vi "Guys Version Host.vi"() -> ()   [LabVIEW 2014]
uses:
  <instrlib>/_niInstr/Streaming/v1/Host/niInstr Streaming v1 Host.lvlib
  <instrlib>/_niInstr/Streaming/v1/Host/Public/Start Finite Stream.vi
  <vilib>/rvi/interface/nirviOpenFPGA/nirviOpenFPGA.xnode
  FPGA Bitfiles/MochiFPGAControl_FPGATarget2_Guysversion_oaYtOet0bo8.lvbitx
  Guys version.vi
  <vilib>/FPGAPlugInAG/PXI-7953R/niLvFpga_Open_PXI-7953R.vi
  <vilib>/rvi/interface/common/dynamic/niFpgaDynamicAddResources.vi
  <vilib>/rvi/interface/nirviMethod/nirviMethod.xnode
  <vilib>/FPGAPlugInAG/Dynamic/niLvFpga_ConfigureFifo_Dynamic.vi
  <vilib>/rvi/errors/niLvFpgaMergeErrorWithErrorCode.vi
  <vilib>/FPGAPlugInAG/Dynamic/niLvFpga_StartFifo_Dynamic.vi
  <instrlib>/_niInstr/Streaming/v1/Host/Public/Wait for Stream.vi
  <vilib>/FPGAPlugInAG/Dynamic/niLvFpga_ReadFifo_Dynamic.vi
  <vilib>/rvi/interface/nirviCloseFPGA/nirviCloseFPGA.xnode
  <vilib>/FPGAPlugInAG/Dynamic/niLvFpga_Close_Dynamic.vi
panel:
  out "error out":errorcluster
  out "samples transferred":u64
  in  "stop":bool
  out "Data":u64[](array[numeric])
  in  "num samples":u64=1000
  in  "Go":bool
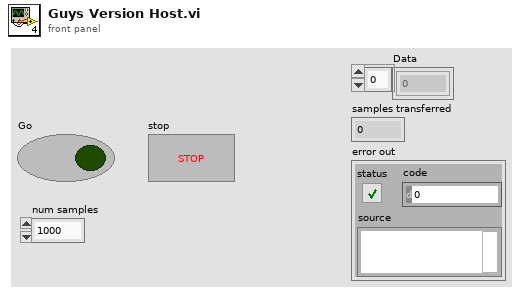
[diagram p1: front panel]
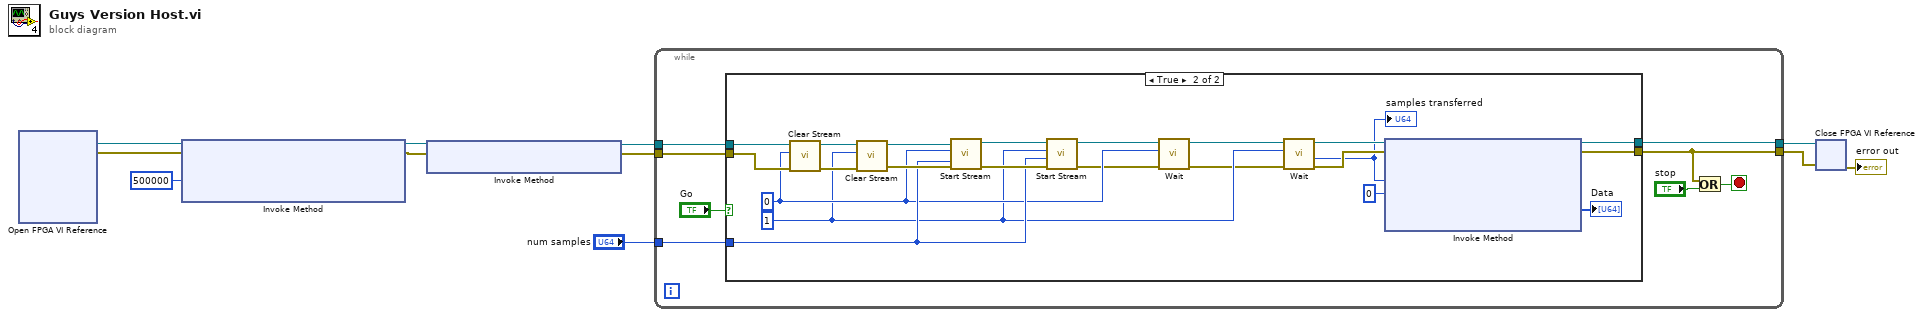
[diagram p0: block diagram]
diagram:
  n1 = xnode "Open FPGA VI Reference"() -> ("FPGA VI Reference Out"=w11:refnum<k20>, "error out"=w9:errorcluster)  [unwired: 2 in]
  n2 = xnode "Invoke Method"("FPGA VI Reference In"=w11, "error in"=w9, "Requested Depth"=u32 500000) -> ("FPGA VI Reference Out"=w8:refnum<k20>, "error out"=w7:errorcluster)  [unwired: 1 out]
  n3 = xnode "Invoke Method"("FPGA VI Reference In"=w8, "error in"=w7) -> ("FPGA VI Reference Out"=w6:refnum<k20>, "error out"=w5:errorcluster)
  n4 = while {
    tunnel: w6 -> [w18]
    tunnel: w5 -> [w17]
    tunnel: "num samples" -> [w16]
    tunnel: [w15] -> w3
    tunnel: [w12] -> w2
    stop <- w13 stop-if-true
    n5 = case shown="True" "Go" {
      tunnel: w18 -> [w21 w43]
      tunnel: w17 -> [w20 w42]
      tunnel: w16 -> [_ w35]
      tunnel: [w20 w23] -> w12
      tunnel: [w21 w22] -> w15
      frame False {
      }
      frame True {
        w30 = 1 ("stream index")
        w33 = 0 ("stream index")
        n6 = call <instrlib>:"Clear Stream.vi"("error in (no error)"=w42, "stream index"=w33, "refnum in"=w43) -> ("error out"=w40:errorcluster, "refnum out"=w41:refnum<k20>)  [unwired: 7 in]
        n7 = call <instrlib>:"Clear Stream.vi"("error in (no error)"=w40, "stream index"=w30, "refnum in"=w41) -> ("error out"=w38:errorcluster, "refnum out"=w39:refnum<k20>)  [unwired: 7 in]
        n8 = call-poly <instrlib>:"Start Stream.vi"("error in (no error)"=w38, "num samples"=w35, "stream index"=w33, "refnum in"=w39) -> ("error out"=w36:errorcluster, "refnum out"=w37:refnum<k20>)  [unwired: 6 in]
        n9 = call-poly <instrlib>:"Start Stream.vi"("error in (no error)"=w36, "num samples"=w35, "stream index"=w30, "refnum in"=w37) -> ("error out"=w32:errorcluster, "refnum out"=w34:refnum<k20>)  [unwired: 6 in]
        n10 = call-poly <instrlib>:"Wait.vi"("error in (no error)"=w32, "stream index"=w33, "refnum in"=w34) -> ("error out"=w29:errorcluster, "refnum out"=w31:refnum<k20>)  [unwired: 5 in, 2 out]
        n11 = call-poly <instrlib>:"Wait.vi"("error in (no error)"=w29, "stream index"=w30, "refnum in"=w31) -> ("error out"=w27:errorcluster, "samples transferred"=w26:u64, "refnum out"=w28:refnum<k20>)  [unwired: 5 in, 1 out]
        "samples transferred" <- w26
        n12 = xnode "Invoke Method"("FPGA VI Reference In"=w28, "error in"=w27, "Number of Elements"=w26, "Timeout (ms)"=0) -> ("FPGA VI Reference Out"=w22:refnum<k20>, "error out"=w23:errorcluster, "Data"=→"Data":u64[])  [unwired: 1 out]
      }
    }
    n13 = Or(x=w12, y="stop") -> (x .or. y?=w13:bool)
  }
  n14 = xnode "Close FPGA VI Reference"("FPGA VI Reference In"=w3, "error in"=w2) -> ("error out"=→"error out":errorcluster)
